vi "DS读数据.vi"() -> ()   [LabVIEW 2010]
panel:
  in  "等待更新值(T)":bool
  in  "stop":bool
  out "超时":bool
  out "循环时间":u32
  out "波形图":dbl[](graph)
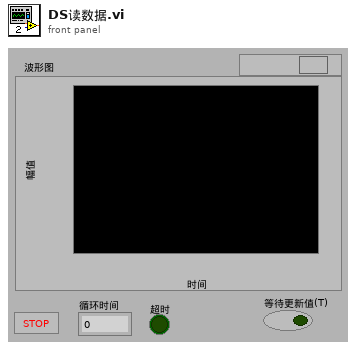
[diagram p1: front panel]
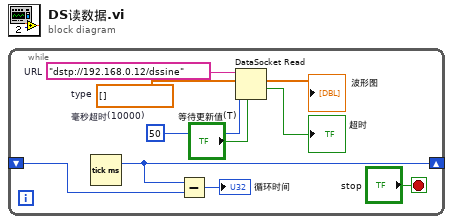
[diagram p0: block diagram]
diagram:
  n1 = while {
    shift-right: [w7] -> _
    shift-left: _ -> [w6]
    stop <- "stop" stop-if-true
    w1 = 50  # 毫秒超时(10000)
    w8 = dbl[] []  # type
    w10 = "dstp://192.168.0.12/dssine"  # URL
    n2 = Tick Count (ms)() -> (millisecond timer value=w7:u32)
    n3 = Subtract(x=w7, y=w6) -> (x-y=→"循环时间":u32)
    n4 = DataSocket Read(6:"等待更新值(T)", 9:w1, 10:w8, 11:w10) -> (1:→"超时":bool, 2:→"波形图":dbl[])  [unwired: 1 in, 5 out]
  }
